vi "EditValue.vi"(8 "error in (no error)":errorcluster, 10 "Bounds":T1, 11 "U32 D Element.lvclass":refnum<class "U32 D Element.lvclass">) -> (0 "error out":errorcluster, 1 "Tabbed out?":bool, 2 "Value changed?":bool, 3 "U32 D Element.lvclass":refnum<class "U32 D Element.lvclass">)   [LabVIEW 2018, in "D Datagrid Library.lvlib" / "U32 D Element.lvclass"]
uses:
  U32 D Element.lvclass
  <vilib>/Utility/miscctls.llb/LVRectTypeDef.ctl
  U32 D Element.lvclass/U32 D Element.ctl
  Read Display mode.vi
panel:
  in  "Value":u32 format="0x%.0x"
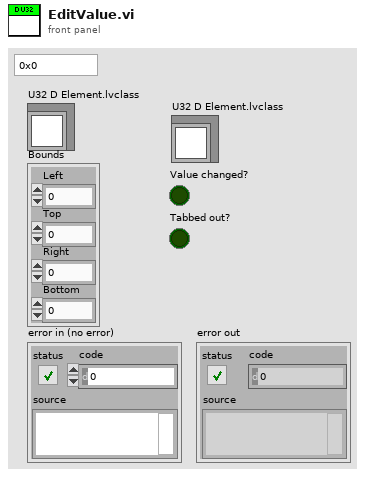
[diagram p1: front panel]
types:
  T1 = typedef "LVRectTypeDef.ctl" = cluster{"Left":i16, "Top":i16, "Right":i16, "Bottom":i16}
  T2 = typedef "D Datagrid Library.lvlib/U32 D Element.lvclass/Display mode.ctl" = enum16{"Standard", "Hex"}
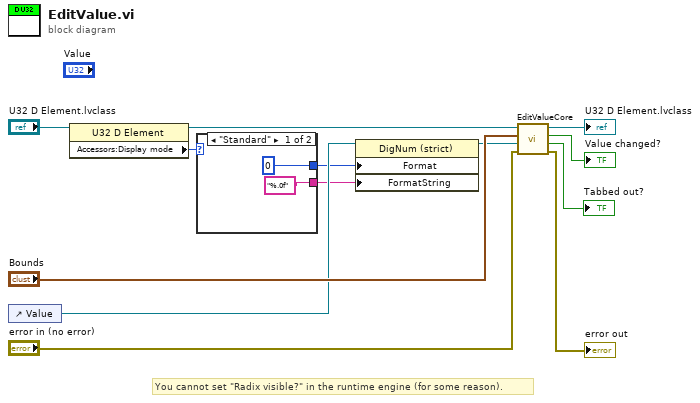
[diagram p0: block diagram]
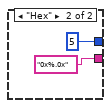
[diagram p2: hidden frame]
diagram:
  # "You cannot set \"Radix visible?\" in the runtime engine (for some reason)."
  n1 = control-ref of="Value"() -> (w5:refnum<vi>)
  n2 = property class="U32 D Element"(reference="U32 D Element.lvclass") -> (reference out=w7:refnum<class "U32 D Element.lvclass">, "Accessors:Display mode"=w6:T2)  [unwired: 1 in, 1 out]
  n3 = case shown="\"Standard\"" w6 {
    tunnel: [u8 0 ("Display Format:Format") u8 5 ("Display Format:Format")] -> w4
    tunnel: ["%.0f" "0x%.0x"] -> w2
    frame "Standard" {
    }
    frame "Hex" {
    }
  }
  n4 = property class="DigNum (strict)"(reference=w5, "Format"=w4, "FormatString"=w2) -> (reference out=w3:refnum<vi>)  [unwired: 1 in, 1 out]
  n5 = call-dynamic "EditValueCore.vi"("error in (no error)"="error in (no error)", "Value field reference"=w3, "Bounds"="Bounds", "DatagridElement in"=w7) -> ("error out"=→"error out":errorcluster, "Tabbed out?"=→"Tabbed out?":bool, "Value changed?"=→"Value changed?":bool, "DatagridElement out"=→"U32 D Element.lvclass":refnum<class "U32 D Element.lvclass">)  [unwired: 4 in]
